vi "solar_voy Write (Handshake).vi"(6 "Suppress Errors? (T)":bool=TRUE, 8 "error in (no error)":errorcluster, 10 "HDR_GUID":string, 11 "Voyager Refnum in":T1) -> (0 "error out":errorcluster, 3 "Voyager Refnum out":T1)   [LabVIEW 2018]
doc: "This returns the registered 'HDR_GUID' and writes the 'HANDSHAKE' packet. The 'HDR_GUID' is registered in a functional global VI that contains the original Target, Packet and Data. If the 'HDR_GUID' is not found, this does nothing."
uses:
  solar_voy_def/solar_voy_def_ctl HANDSHAKE.ctl
  solar_voy_ctl Voyager Refnum.ctl
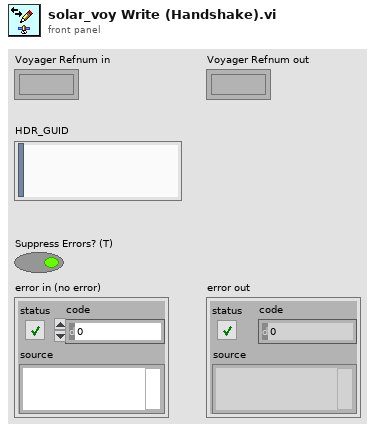
[diagram p1: front panel]
types:
  T1 = typedef "solar_voy_ctl Voyager Refnum.ctl" = refnum<k1>
  T2 = typedef "solar_voy_def_ctl HANDSHAKE.ctl" = cluster{"ORIGIN":enum8{"RMT", "LCL"}, "STATUS,s=OK,ERROR":bool, "CODE":i32, "TIME_SECONDS":u32, "TIME_MICROSECONDS":u32, "DATA,t=BLOCK":string}
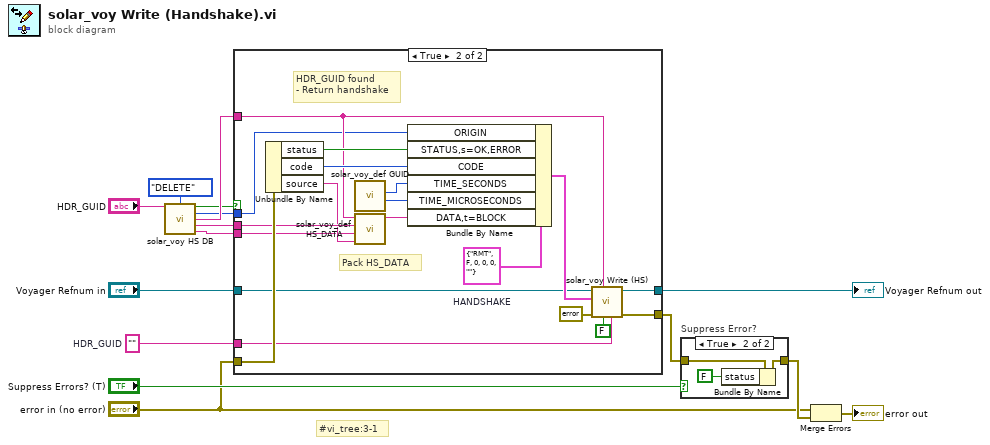
[diagram p0: block diagram]
diagram:
  w9 = ""  # HDR_GUID
  # "#vi_tree:3-1"
  n1 = call "solar_voy HS DB.vi"("HDR_GUID"="HDR_GUID", "Action"=enum8{"DELETE", "ADD", "CLEAR"}."DELETE") -> ("Exists?"=w2:bool, "ORIGIN out"=w1:enum8{"RMT", "LCL"}, "TARGET out"=w6:string, "PACKET out"=w5:string, "DATA out"=w4:string)  [unwired: 9 in]
  n2 = case shown="True" w2 {
    tunnel: [_ w35] -> w12
    tunnel: [w16 w34] -> w11
    tunnel: "error in (no error)" -> [_ w30]
    tunnel: "Voyager Refnum in" -> [w16 w24]
    tunnel: w6 -> [_ w23]
    tunnel: w5 -> [_ w22]
    tunnel: w9 -> [_ w20]
    tunnel: w4 -> [_ w19]
    tunnel: w1 -> [_ w17]
    frame False {
      # "HDR_GUID not found\n- Do nothing"
    }
    frame True {
      w32 = T2 {"ORIGIN"=enum."RMT", "STATUS,s=OK,ERROR"=FALSE, "CODE"=0, "TIME_SECONDS"=0, "TIME_MICROSECONDS"=0, "DATA,t=BLOCK"=""}  # HANDSHAKE
      # "HDR_GUID found\n- Return handshake"
      # "Pack HS_DATA"
      n3 = Unbundle By Name(w30) -> ("status"=w29:bool, "code"=w28:i32, "source"=w21:string)
      n4 = call "solar_voy_def GUID.vi"() -> ("TIME_MICROSECONDS"=w26:u32, "TIME_SECONDS"=w27:u32)  [unwired: 8 in, 2 out]
      n5 = call "solar_voy_def HS_DATA.vi"("Error Source"=w21, "PACKET_DATA"=w19, "PACKET"=w22, "TARGET"=w23) -> ("HS_DATA"=w25:string)  [unwired: 7 in]
      n6 = Bundle By Name(cluster=w32, "ORIGIN"=w17, "STATUS,s=OK,ERROR"=w29, "CODE"=w28, "TIME_SECONDS"=w27, "TIME_MICROSECONDS"=w26, "DATA,t=BLOCK"=w25) -> (w31:T2)
      n7 = call "solar_voy Write (HS).vi"("HDR_GUID"=w20, "Suppress Errors? (T)"=FALSE, "TARGET"=w23, "error in (no error)"=errorcluster {"status"=FALSE, "code"=0, "source"=""}, "HANDSHAKE"=w31, "Voyager Refnum in"=w24) -> ("error out"=w35:errorcluster, "Voyager Refnum out"=w34:T1)  [unwired: 4 in]
    }
  }
  "Voyager Refnum out" <- w11
  n8 = case "Suppress Error?" shown="True" "Suppress Errors? (T)" {
    tunnel: w12 -> [w36 w39]
    tunnel: [w36 w38] -> w14
    frame False {
    }
    frame True {
      n9 = Bundle By Name(cluster=w39, "status"=FALSE) -> (w38:errorcluster)
    }
  }
  n10 = Merge Errors("error in (no error)", w14) -> (→"error out":errorcluster)
